vi "demo_Nigel Enhancements in 2026 Q3.vi"(11 "Stop Demo":refnum<user-event>) -> ()   [LabVIEW 2020]
panel:
  # "LabVIEW 2026 Q3 - Nigel AI Updates\n\n- You can prompt Nigel to generate VIs.\n- You can use the Add File to Context button to pass text files and VIs to Nigel.\n- For eligible VIs, Nigel will clean up the front panels with Edit » Clean Up Panel.\n- Nigel now allows you to select the AI model used to answer your queries.\n- Nigel now supports connecting to Model Context Protocol (MCP) servers."
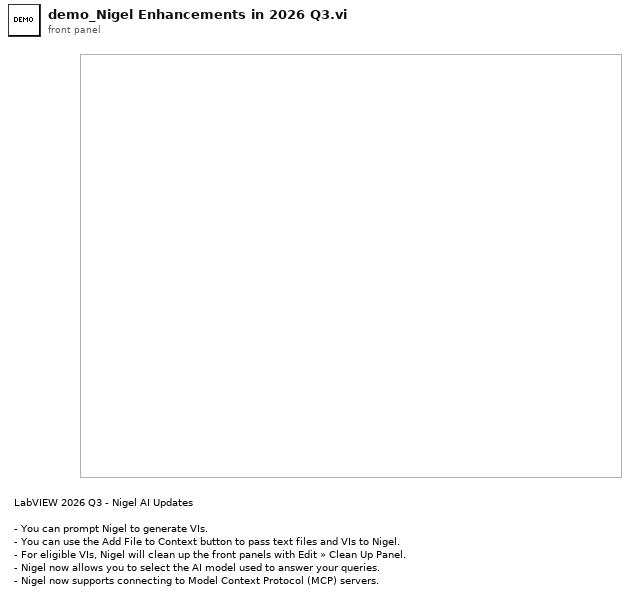
[diagram p1: front panel]
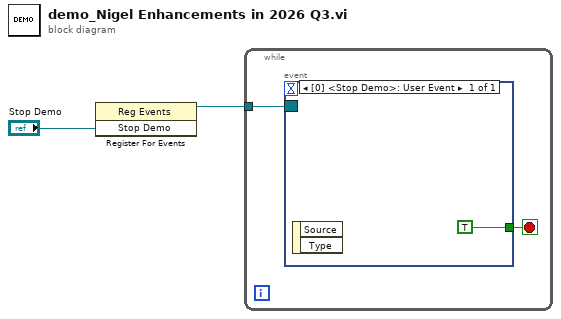
[diagram p0: block diagram]
diagram:
  n1 = register-events("Stop Demo") -> (reference out=w1:refnum<event-registration>)  [unwired: 2 in, 1 out]
  n2 = while {
    tunnel: w1 -> [w4]
    stop <- w3 stop-if-true
    n3 = event shown="[0] <Stop Demo>: User Event" {
      selector: w4 -> [_]
      dyn-events: _ -> [_]
      timeout: _ -> [_]
      tunnel: [TRUE] -> w3
      event User Event {
        n4 = event-data() -> ()  [unwired: 1 in, 2 out]
      }
    }
  }
